vi "ILABW_CaseHandlerNoPath.vi"(2 "data":string, 3 "action":string) -> (0 "errorOut":string, 1 "response":string)   [LabVIEW 2012]
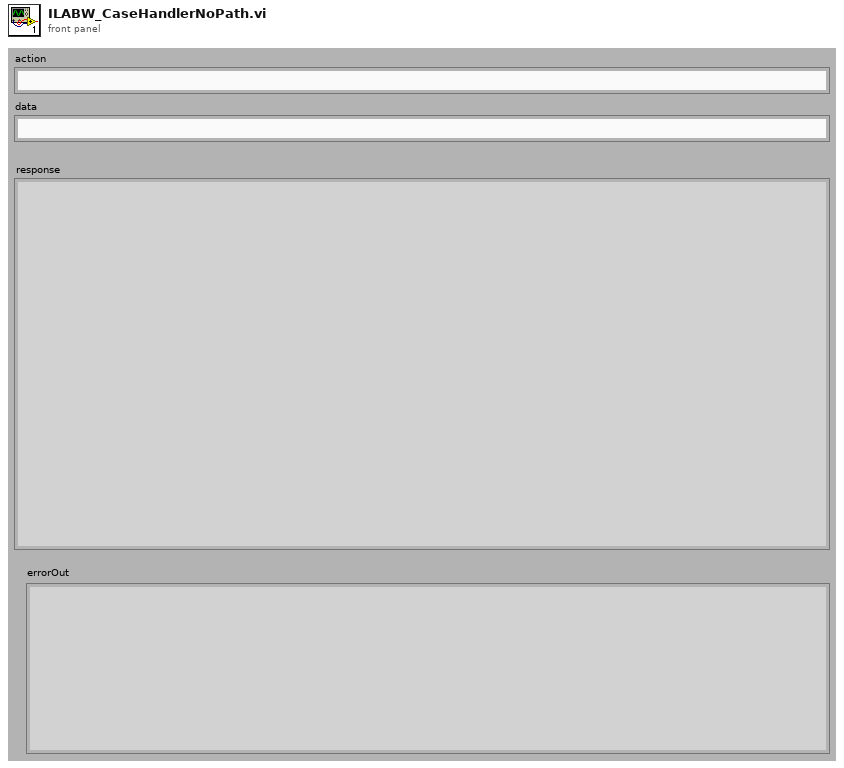
[diagram p1: front panel]
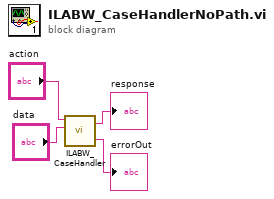
[diagram p0: block diagram]
diagram:
  n1 = call "ILABW_CaseHandler.vi"("data"="data", "action"="action") -> ("errorOut"=→"errorOut":string, "response"=→"response":string)  [unwired: 2 in]
